vi "EMS Device Activate Status.vi"(6 "error string":string, 8 "error in (no error)":errorcluster, 9 "Status":T1, 10 "IED Name":string, 11 "Master Controller in":refnum<class "Master Controller.lvclass">) -> (0 "error out":errorcluster, 3 "Master Controller out":refnum<class "Master Controller.lvclass">)   [LabVIEW 2015, in "Master Controller Core.lvlib" / "Master Controller.lvclass"]
uses:
  Master Controller.lvclass
  SCADA Core/SCADA Abstract Messages/Device Action Status Msg/Device Action Status.ctl
  Communications/SCADA Communcations Actor/SCADA Communications/Controls/EMS Message Cluster.ctl
  Master Controller.lvclass/Master Controller.ctl
  Communications/SCADA Communcations Actor/SCADA Communications Messages/Transmit EMS Message Msg/Transmit EMS Message Msg.lvclass/Transmit EMS Message Msg.ctl
  <vilib>/ActorFramework/Message Enqueuer/Message Enqueuer.lvclass/Message Enqueuer.ctl
  <vilib>/ActorFramework/Message Enqueuer/Enqueue.vi
  <vilib>/ActorFramework/Message Priority Queue/Priority Enqueue.vi
  Communications/SCADA Communcations Actor/SCADA Communications Messages/Transmit EMS Message Msg/Transmit EMS Message Msg.lvclass
  Utilities/Message Strings.llb/Message String Utilities.lvlib
  Communications/SCADA Communcations Actor/SCADA Communications/SCADA Communications.lvclass
  SCADA Core/SCADA Abstract Messages/Device Action Status Msg/Device Action Status Msg.lvclass
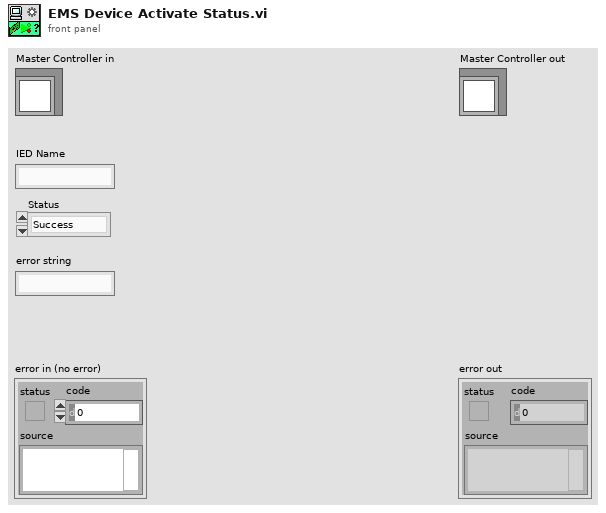
[diagram p1: front panel]
types:
  T1 = typedef "SCADA Core.lvlib/Device Action Status Msg.lvclass/Device Action Status.ctl" = enum16{"Success", "Failure"}
  T2 = typedef "SCADA Communcations Actor.lvlib/SCADA Communications.lvclass/EMS Message Cluster.ctl" = cluster{"Name":string, "Content":string}
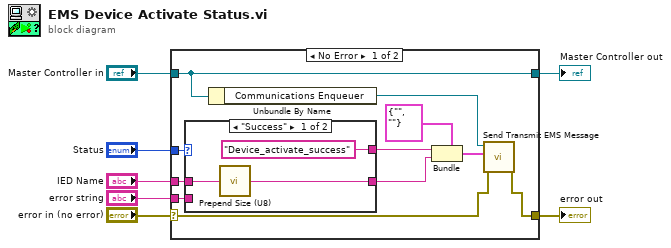
[diagram p0: block diagram]
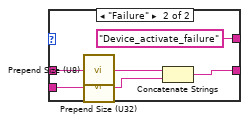
[diagram p2: hidden frame]
diagram:
  n1 = case shown="No Error" "error in (no error)" {
    selector: "error in (no error)" -> [w13 w29]
    tunnel: [w12 w29] -> w6
    tunnel: [w17 w28] -> w4
    tunnel: "Master Controller in" -> [w17 w28]
    tunnel: "IED Name" -> [w10 _]
    tunnel: "Status" -> [w18 _]
    tunnel: "error string" -> [w9 _]
    frame No Error {
      n2 = case shown="\"Success\"" w18 {
        tunnel: ["Device_activate_success" ("Name") "Device_activate_failure" ("Name")] -> w11
        tunnel: w10 -> [w20 w26]
        tunnel: w9 -> [_ w25]
        tunnel: [w19 w22] -> w8
        frame "Success" {
          n3 = call "Prepend Size (U8).vi"("String in"=w20) -> ("String out"=w19:string)
        }
        frame "Failure" {
          n4 = call "Prepend Size (U8).vi"("String in"=w26) -> ("String out"=w24:string)
          n5 = call "Prepend Size (U32).vi"("String in"=w25) -> ("String out"=w23:string)
          n6 = Concatenate Strings(w24, w23) -> (w22:string)
        }
      }
      n7 = Unbundle By Name(w17) -> ("Communications Enqueuer"=w15:refnum<class "Message Enqueuer.lvclass">)
      n8 = Bundle(cluster=T2 {"Name"="", "Content"=""} ("Message"), "Name"=w11, "Content"=w8) -> (w14:T2)
      n9 = call "Send Transmit EMS Message.vi"("error in (no error)"=w13, "Message"=w14, "Message Enqueuer"=w15) -> ("error out"=w12:errorcluster)  [unwired: 7 in, 1 out]
    }
    frame Error {
    }
  }
  "error out" <- w6
  "Master Controller out" <- w4
